vi "Spectral Analysis.vi"() -> ()   [LabVIEW 2015]
uses:
  <vilib>/Analysis/4window.llb/windowTd.ctl
  <vilib>/measure/maspectr.llb/Power Spectrum and PSD Export Mode.ctl
  <vilib>/Analysis/5stat.llb/RMS (DBL).vi
  <vilib>/Utility/file.llb/Read From Spreadsheet File (DBL).vi
  <vilib>/measure/maspectr.llb/FFT Spectrum (Mag-Phase) for 1 Chan.vi
  <vilib>/measure/maspectr.llb/FFT Power Spectrum and PSD for 1 Chan.vi
  <vilib>/measure/NI_MAPro.lvlib
  <vilib>/Analysis/NI_AALPro.lvlib
  <vilib>/Analysis/NI_AALBase.lvlib
panel:
  in  "dt":dbl=0.002 format="%#_13g"
  out "RMS Value 2":dbl
  out "Displacement":dbl[](graph)
  out "RMS Value":dbl
  in  "View":T1={"dB On (F)"=TRUE, "Unwrap Phase (F)"=TRUE, "Convert to Degree (F)"=FALSE}
  in  "window":T2=6 items=["Rectangle"=0, "Hanning"=1, "Hamming"=2, "Blackman-Harris"=3, "Exact Blackman"=4, "Blackman"=5, "Flat Top"=6, "4 Term B-Harris "=7, "7 Term B-Harris"=8, "Low Sidelobe"=9, "Blackman Nuttall"=11, "Triangle"=30, "Bartlett-Hanning"=31, "Bohman"=32, "Parzen"=33, "Welch"=34, "Kaiser"=60, "Dolph-Chebyshev"=61, "Gaussian"=62]
  in  "averaging parameters":T3={"averaging mode"=enum."No averaging", "weighting mode"=enum."Exponential", "number of averages"=10} {"number of averages" min=1}
  in  "Measurement Type":T4(ring)
  out "Sample Size":i32
  out "Rate - Windowed":waveform(dbl)(graph)
  out "Phase":cluster{"f0":dbl, "df":dbl, "phase":dbl[]}(graph)
  out "Amplitude":cluster{"f0":dbl, "df":dbl, "magnitude":dbl[]}(graph)
  in  "Select Column":i32
  in  "file path (dialog if empty)":path
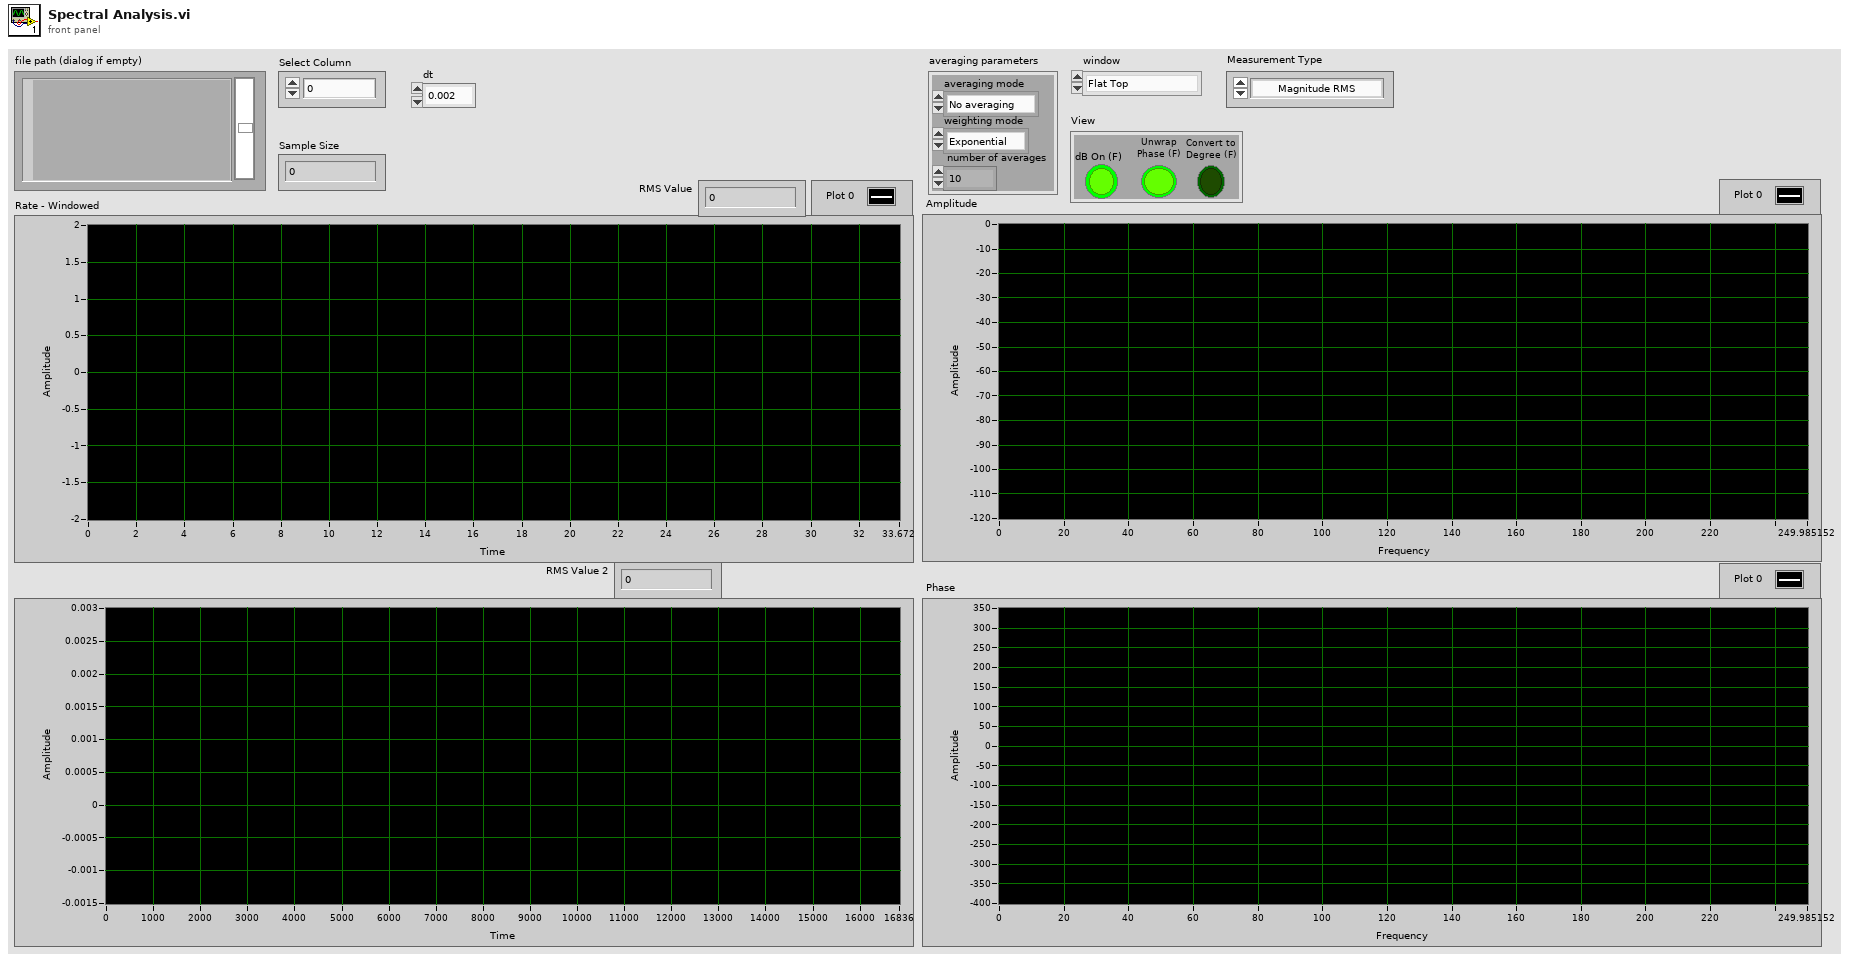
[diagram p1: front panel]
types:
  T1 = cluster{"dB On (F)":bool, "Unwrap Phase (F)":bool, "Convert to Degree (F)":bool}
  T2 = typedef "NI_AALPro.lvlib/windowTd.ctl" = u32
  T3 = cluster{"averaging mode":enum16{"No averaging", "Vector averaging", "RMS averaging", "Peak hold"}, "weighting mode":enum16{"Linear", "Exponential"}, "number of averages":u32}
  T4 = enum16{"Magnitude RMS", "Power Spectrum", "Power Spectral Density"}
  T5 = typedef "NI_MAPro.lvlib/Power Spectrum and PSD Export Mode.ctl" = u16
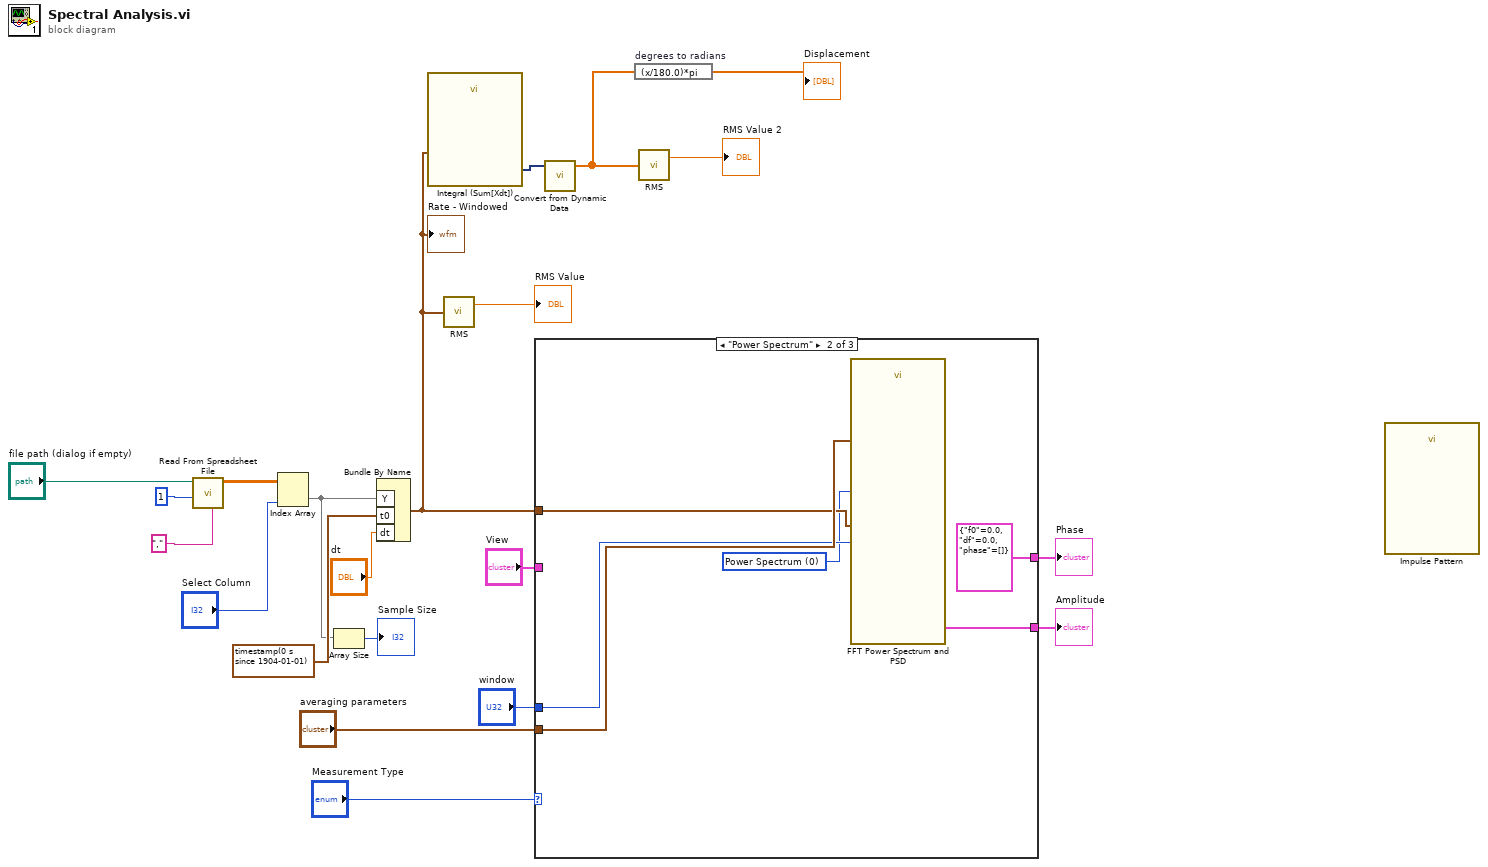
[diagram p0: block diagram]
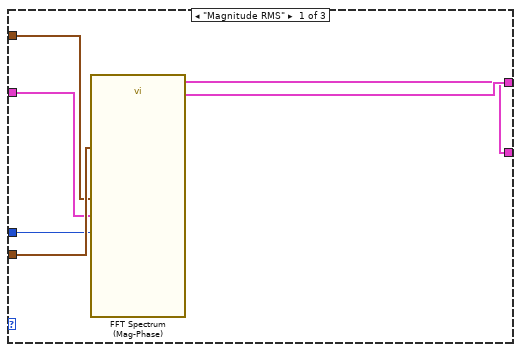
[diagram p2: hidden frame]
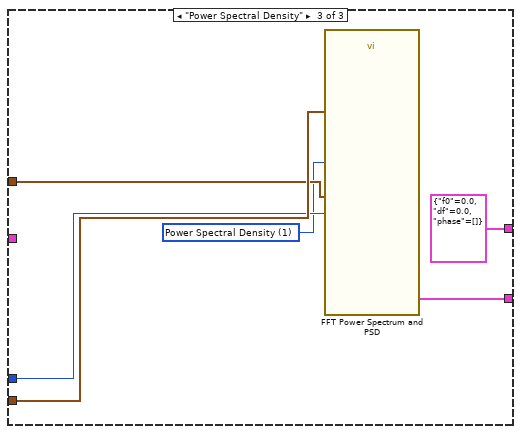
[diagram p3: hidden frame]
diagram:
  n1 = call-poly <vilib>:"Read From Spreadsheet File.vi"("delimiter (\\t)"="," ("delimiter (\\t)"), "start of read offset (chars.:0)"=1, "file path (dialog if empty)"="file path (dialog if empty)") -> ("all rows"=w21:dbl[][])  [unwired: 4 in, 4 out]
  n2 = Index Array(array=w21, index (col)="Select Column") -> (element=w6:dbl[])  [unwired: 1 in]
  n3 = Array Size(array=w6) -> (size(s)=→"Sample Size":i32)
  n4 = Bundle By Name("Y"=w6, "t0"=timestamp(0 s since 1904-01-01), "dt"="dt") -> (w4:waveform(dbl))  [unwired: 1 in]
  "Rate - Windowed" <- w4
  n5 = call "Integral (Sum[Xdt])"("Signals"=w4) -> ("Result"=w3:dynamicdata)  [unwired: 5 in, 1 out]
  n6 = call-poly <vilib>:"RMS.vi"("X"=w4) -> ("rms value"=→"RMS Value":dbl)  [unwired: 1 out]
  n7 = case shown="\"Power Spectrum\"" "Measurement Type" {
    tunnel: w4 -> [w22 w31 w38]
    tunnel: "averaging parameters" -> [w27 w32 w39]
    tunnel: "window" -> [w25 w30 w36]
    tunnel: [w24 cluster{"f0":dbl, "df":dbl, "phase":dbl[]} {"f0"=0.0, "df"=0.0, "phase"=[]} ("phase") cluster{"f0":dbl, "df":dbl, "phase":dbl[]} {"f0"=0.0, "df"=0.0, "phase"=[]} ("phase")] -> w10
    tunnel: "View" -> [w26 _ _]
    tunnel: [w23 w28 w34] -> w8
    frame "Magnitude RMS" {
      n8 = call-poly <vilib>:"FFT Spectrum (Mag-Phase).vi"("averaging parameters"=w27, "view"=w26, "window"=w25, "time signal"=w22) -> ("phase"=w24:cluster{"f0":dbl, "df":dbl, "phase":dbl[]}, "magnitude"=w23:cluster{"f0":dbl, "df":dbl, "magnitude":dbl[]})  [unwired: 3 in, 3 out]
    }
    frame "Power Spectrum" {
      w29 = T5 0 items=["Power Spectrum", "Power Spectral Density"] ("export mode")
      n9 = call-poly <vilib>:"FFT Power Spectrum and PSD.vi"("export mode"=w29, "averaging parameters"=w32, "window"=w30, "time signal"=w31) -> ("Power Spectrum / PSD"=w28:cluster{"f0":dbl, "df":dbl, "magnitude":dbl[]})  [unwired: 4 in, 3 out]
    }
    frame "Power Spectral Density" {
      w35 = T5 1 items=["Power Spectrum", "Power Spectral Density"] ("export mode")
      n10 = call-poly <vilib>:"FFT Power Spectrum and PSD.vi"("export mode"=w35, "averaging parameters"=w39, "window"=w36, "time signal"=w38) -> ("Power Spectrum / PSD"=w34:cluster{"f0":dbl, "df":dbl, "magnitude":dbl[]})  [unwired: 4 in, 3 out]
    }
  }
  "Amplitude" <- w8
  "Phase" <- w10
  n11 = call "Convert from Dynamic Data"("Dynamic Data Type"=w3) -> ("Array"=w2:dbl[])  [unwired: 3 in]
  n12 = expression code="(x/180.0)*pi" "degrees to radians"(w2) -> (→"Displacement":dbl[])
  n13 = call-poly <vilib>:"RMS.vi"("X"=w2) -> ("rms value"=→"RMS Value 2":dbl)  [unwired: 1 out]
  n14 = call <vilib>:"Impulse Pattern.vi"() -> ()  [unwired: 3 in, 2 out]
